vi "convertNumberColorToLetter.vi"() -> (11 "String":string)   [LabVIEW 2019]
uses:
  <vilib>/regexp/Match Regular Expression.xnode
panel:
  out "spreadsheet string":string
  in  "Array":string[](array[string])
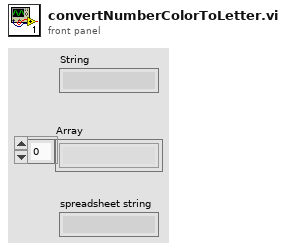
[diagram p1: front panel]
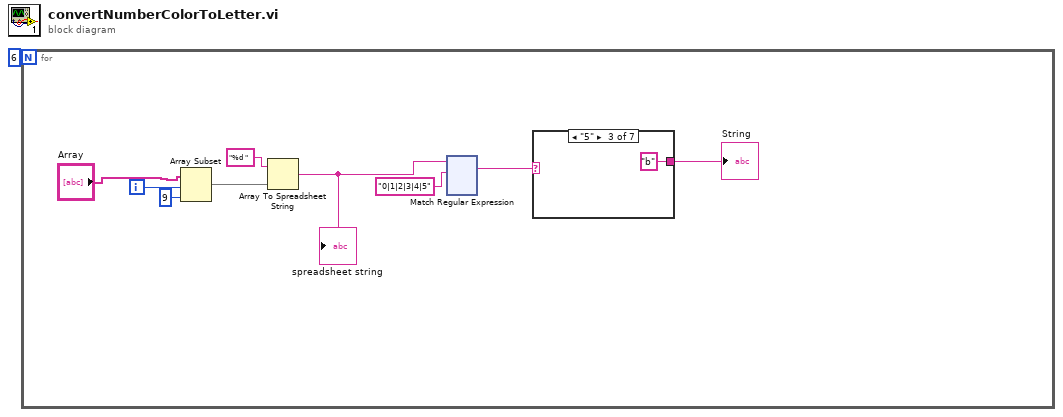
[diagram p0: block diagram]
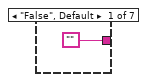
[diagram p2: hidden frame]
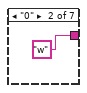
[diagram p3: hidden frame]
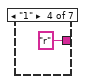
[diagram p4: hidden frame]
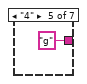
[diagram p5: hidden frame]
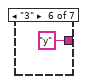
[diagram p6: hidden frame]
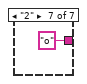
[diagram p7: hidden frame]
diagram:
  n1 = for {
    N: 6 -> [_]
    i -> [w5]
    n2 = Array Subset(array="Array", index=w5, length=9) -> (w2:string[])
    n3 = Array To Spreadsheet String(array=w2, 3:"%d " ("format string")) -> (spreadsheet string=w9:string)  [unwired: 1 in]
    "spreadsheet string" <- w9
    n4 = xnode "Match Regular Expression"("input string"=w9, "regular expression"="0|1|2|3|4|5" ("input string")) -> ("whole match"=w6:string)  [unwired: 4 in, 4 out]
    n5 = case shown="\"5\"" w6 {
      tunnel: ["" "w" "b" "r" "g" "y" "o"] -> w7
      frame "False", Default {
      }
      frame "0" {
      }
      frame "5" {
      }
      frame "1" {
      }
      frame "4" {
      }
      frame "3" {
      }
      frame "2" {
      }
    }
    "String" <- w7
  }
